vi "EMGain.vi"() -> ()   [LabVIEW 2018]
uses:
  D:/SVN/PM/sdk/AppSamples/LabVIEWSamples/trunk/Release/2018/Dependencies/PVCamNET.dll
  Dependencies/PVCamNET.dll
panel:
  in  "EM Gain Scrollbar":i32(c297)
  in  "Exposure":u32
  in  "?":bool
  out "EM Gain":dbl
  in  "Port":string(combo)
  in  "?":bool
  in  "Gain":string(combo)
  in  "?":bool
  in  "?":bool
  # "EMGain.vi\n\nDescription:\nThis sample code lets the user control the EM Gain.\n\nSteps to run:\n1. Click \"Run\"\n2. Click \"START\"\n3. Update exposure.\n4. Select Port with EM gain enabled\n5. Increase EM Gain\n6. Click \"Start Live\"\n7. Click \"Stop Live\"\n8. Click \"STOP\"\n\nNote: For cameras don't support EM gain this VI shouldn't be run.\nAlso the focus of this VI is to use EM Gain, not Gain and thus Gain is disabled with this VI."
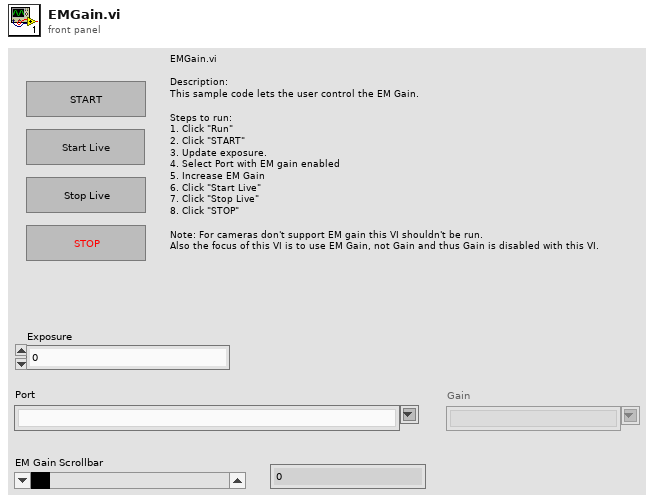
[diagram p1: front panel]
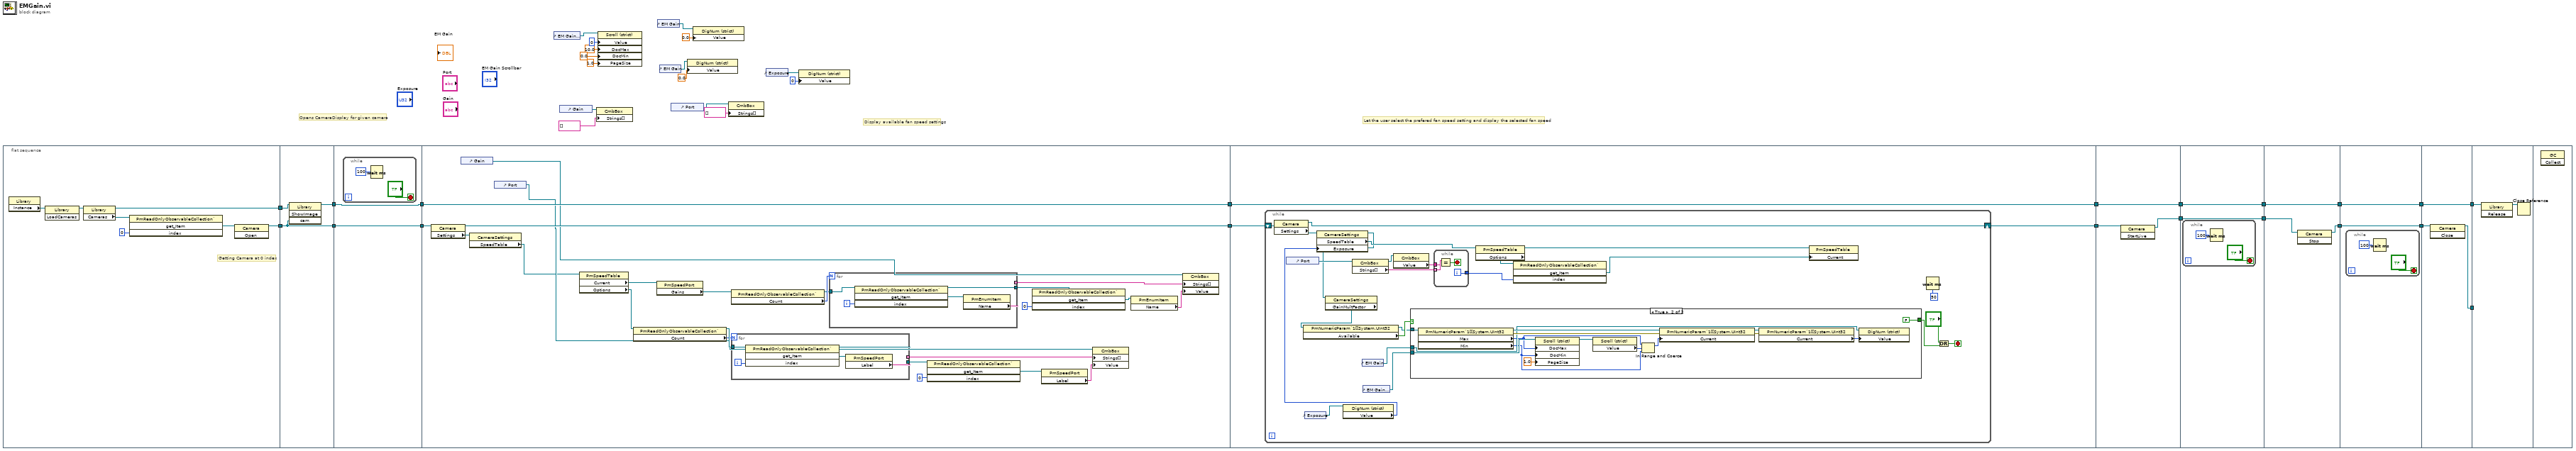
[diagram p0: block diagram]
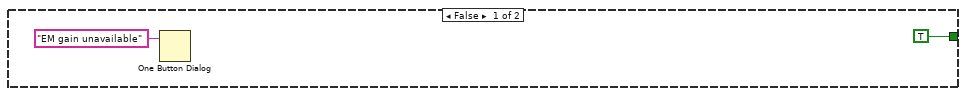
[diagram p2: hidden frame]
diagram:
  # "Let the user select the prefered fan speed setting and display the selected fan speed"
  # "Display available fan speed settings"
  # "Opens CameraDisplay for given camera"
  n1 = flat-sequence {
    tunnel: [w38] -> w35
    tunnel: [w39] -> w34
    tunnel: w35 -> [w45]
    tunnel: w34 -> [w44]
    tunnel: [w44] -> w33
    tunnel: [w43] -> w32
    tunnel: w33 -> [w47]
    tunnel: [w47] -> w30
    tunnel: w32 -> [w46]
    tunnel: [w46] -> w31
    tunnel: [w73] -> w25
    tunnel: [w72] -> w24
    tunnel: w31 -> [w72]
    tunnel: w30 -> [w71]
    tunnel: w25 -> [w86]
    tunnel: [w84] -> w17
    tunnel: w24 -> [w85]
    tunnel: [w85] -> w16
    tunnel: w17 -> [w133]
    tunnel: w16 -> [w134]
    tunnel: [w134] -> w13
    tunnel: [w132] -> w10
    tunnel: w13 -> [w136]
    tunnel: [w136] -> w12
    tunnel: [w135] -> w11
    tunnel: w10 -> [w135]
    tunnel: [w140] -> w15
    tunnel: w12 -> [w141]
    tunnel: [w141] -> w14
    tunnel: w11 -> [w139]
    tunnel: w15 -> [w143]
    tunnel: [w143] -> w27
    tunnel: [w142] -> w26
    tunnel: w14 -> [w142]
    tunnel: w27 -> [w148]
    tunnel: w26 -> [w146]
    tunnel: [w147] -> w29
    tunnel: [w146] -> w28
    tunnel: w29 -> [_]
    tunnel: w28 -> [w150]
    frame #0 {
      # "Getting Camera at 0 index"
      n2 = property class="Library"() -> ("Instance"=w37:refnum<k24>)  [unwired: 2 in, 2 out]
      n3 = invoke class="Library" method="LoadCameras"(reference=w37) -> (reference out=w36:refnum<k24>)  [unwired: 2 in, 2 out]
      n4 = property class="Library"(reference=w36) -> (reference out=w38:refnum<k24>, "Cameras"=w42:refnum<k24>)  [unwired: 1 in, 1 out]
      n5 = invoke class="PmReadOnlyObservableCollection`" method="get_Item"(reference=w42, "index"=0) -> ("get_Item"=w40:refnum<k24>)  [unwired: 2 in, 3 out]
      n6 = invoke class="Camera" method="Open"(reference=w40) -> (reference out=w39:refnum<k24>)  [unwired: 2 in, 2 out]
    }
    frame #1 {
      n7 = invoke class="Library" method="ShowImage"(reference=w45, "cam"=w44) -> (reference out=w43:refnum<k24>)  [unwired: 2 in, 3 out]
    }
    frame #2 {
      n8 = while {
        stop <- "?" stop-if-true
        n9 = Wait (ms)(milliseconds to wait=u32 100) -> ()  [unwired: 1 out]
      }
    }
    frame #3 {
      n10 = property class="Camera"(reference=w71) -> (reference out=w73:refnum<k24>, "Settings"=w70:refnum<k24>)  [unwired: 1 in, 1 out]
      n11 = control-ref of="Gain"() -> (w52:refnum<vi>)
      n12 = property class="CameraSettings"(reference=w70) -> ("SpeedTable"=w50:refnum<k24>)  [unwired: 1 in, 2 out]
      n13 = control-ref of="Port"() -> (w51:refnum<vi>)
      n14 = property class="PmSpeedTable"(reference=w50) -> ("Current"=w69:refnum<k24>, "Options"=w62:refnum<k24>)  [unwired: 1 in, 2 out]
      n15 = property class="PmReadOnlyObservableCollection`"(reference=w62) -> (reference out=w61:refnum<k24>, "Count"=w60:i32)  [unwired: 1 in, 1 out]
      n16 = property class="PmSpeedPort"(reference=w69) -> ("Gains"=w68:refnum<k24>)  [unwired: 1 in, 2 out]
      n17 = property class="PmReadOnlyObservableCollection`"(reference=w68) -> (reference out=w66:refnum<k24>, "Count"=w67:i32)  [unwired: 1 in, 1 out]
      n18 = for {
        N: w60 -> [_]
        tunnel: w61 -> [w78]
        tunnel: [w76] -> w56
        tunnel: [w74] -> w59 mode=indexing
        i -> [w77]
        n19 = invoke class="PmReadOnlyObservableCollection`" method="get_Item"(reference=w78, "index"=w77) -> (reference out=w76:refnum<k24>, "get_Item"=w75:refnum<k24>)  [unwired: 2 in, 2 out]
        n20 = property class="PmSpeedPort"(reference=w75) -> ("Label"=w74:string)  [unwired: 1 in, 2 out]
      }
      n21 = for {
        N: w67 -> [_]
        tunnel: w66 -> [w83]
        tunnel: [w80] -> w64
        tunnel: [w79] -> w63 mode=indexing
        i -> [w82]
        n22 = invoke class="PmReadOnlyObservableCollection`" method="get_Item"(reference=w83, "index"=w82) -> (reference out=w80:refnum<k24>, "get_Item"=w81:refnum<k24>)  [unwired: 2 in, 2 out]
        n23 = property class="PmEnumItem"(reference=w81) -> ("Name"=w79:string)  [unwired: 1 in, 2 out]
      }
      n24 = invoke class="PmReadOnlyObservableCollection`" method="get_Item"(reference=w56, "index"=0) -> ("get_Item"=w57:refnum<k24>)  [unwired: 2 in, 3 out]
      n25 = invoke class="PmReadOnlyObservableCollection`" method="get_Item"(reference=w64, "index"=0) -> ("get_Item"=w65:refnum<k24>)  [unwired: 2 in, 3 out]
      n26 = property class="PmSpeedPort"(reference=w57) -> ("Label"=w58:string)  [unwired: 1 in, 2 out]
      n27 = property class="CmbBox"(reference=w51, "Strings[]"=w59, "Value"=w58) -> ()  [unwired: 1 in, 2 out]
      n28 = property class="PmEnumItem"(reference=w65) -> ("Name"=w55:string)  [unwired: 1 in, 2 out]
      n29 = property class="CmbBox"(reference=w52, "Strings[]"=w63, "Value"=w55) -> ()  [unwired: 1 in, 2 out]
    }
    frame #4 {
      n30 = while {
        shift-right: [w108] -> w84
        shift-left: w86 -> [w109]
        stop <- w90 stop-if-true
        n31 = property class="Camera"(reference=w109) -> (reference out=w108:refnum<k24>, "Settings"=w110:refnum<k24>)  [unwired: 1 in, 1 out]
        n32 = control-ref of="Port"() -> (w99:refnum<vi>)
        n33 = control-ref of="Exposure"() -> (w89:refnum<vi>)
        n34 = property class="DigNum (strict)"(reference=w89) -> ("Value"=w88:u32)  [unwired: 1 in, 2 out]
        n35 = property class="CameraSettings"(reference=w110, "Exposure"=w88) -> (reference out=w97:refnum<k24>, "SpeedTable"=w100:refnum<k24>)  [unwired: 1 in, 1 out]
        n36 = property class="CameraSettings"(reference=w97) -> ("GainMultFactor"=w96:refnum<k24>)  [unwired: 1 in, 2 out]
        n37 = property class="PmNumericParam`1[[System.UInt32"(reference=w96) -> (reference out=w94:refnum<k24>, "Available"=w95:bool)  [unwired: 1 in, 1 out]
        n38 = property class="CmbBox"(reference=w99) -> (reference out=w102:refnum<vi>, "Strings[]"=w106:string[])  [unwired: 1 in, 1 out]
        n39 = control-ref of="EM Gain"() -> (w93:refnum<vi>)
        n40 = control-ref of="EM Gain Scrollbar"() -> (w87:refnum<vi>)
        n41 = property class="CmbBox"(reference=w102) -> ("Value"=w101:string)  [unwired: 1 in, 2 out]
        n42 = case shown="True" w95 {
          tunnel: w94 -> [_ w127]
          tunnel: w93 -> [_ w119]
          tunnel: [TRUE FALSE] -> w91
          tunnel: w87 -> [_ w118]
          frame False {
            n43 = One Button Dialog(message="EM gain unavailable") -> ()  [unwired: 1 in, 1 out]
          }
          frame True {
            n44 = property class="PmNumericParam`1[[System.UInt32"(reference=w127) -> (reference out=w125:refnum<k24>, error out=w123:errorcluster, "Max"=w117:u32, "Min"=w116:u32)  [unwired: 1 in]
            n45 = property class="Scroll (strict)"(reference=w118, "DocMax"=w117, "DocMin"=w116, "PageSize"=1.0 ("Page Size")) -> (reference out=w114:refnum<vi>)  [unwired: 1 in, 1 out]
            n46 = property class="Scroll (strict)"(reference=w114) -> ("Value"=w113:i32)  [unwired: 1 in, 2 out]
            n47 = In Range and Coerce(upper limit=w117, x=w113, lower limit=w116) -> (coerced(x)=w126:u32)  [unwired: 1 out]
            n48 = property class="PmNumericParam`1[[System.UInt32"(reference=w125, error in=w123, "Current"=w126) -> (reference out=w124:refnum<k24>, error out=w122:errorcluster)
            n49 = property class="PmNumericParam`1[[System.UInt32"(reference=w124, error in=w122) -> ("Current"=w121:u32)  [unwired: 2 out]
            n50 = property class="DigNum (strict)"(reference=w119, "Value"=w121) -> ()  [unwired: 1 in, 2 out]
          }
        }
        n51 = while {
          tunnel: w106 -> [w131] mode=indexing
          tunnel: [w129] -> w104
          tunnel: w101 -> [w128]
          i -> [w129]
          stop <- w130 stop-if-true
          n52 = Equal?(x=w131, y=w128) -> (x = y?=w130:bool)
        }
        n53 = property class="PmSpeedTable"(reference=w100) -> (reference out=w103:refnum<k24>, "Options"=w105:refnum<k24>)  [unwired: 1 in, 1 out]
        n54 = invoke class="PmReadOnlyObservableCollection`" method="get_Item"(reference=w105, "index"=w104) -> ("get_Item"=w98:refnum<k24>)  [unwired: 2 in, 3 out]
        n55 = property class="PmSpeedTable"(reference=w103, "Current"=w98) -> ()  [unwired: 1 in, 2 out]
        n56 = Wait (ms)(milliseconds to wait=u32 50) -> ()  [unwired: 1 out]
        n57 = Or(x="?", y=w91) -> (x .or. y?=w90:bool)
      }
    }
    frame #5 {
      n58 = invoke class="Camera" method="StartLive"(reference=w133) -> (reference out=w132:refnum<k24>)  [unwired: 2 in, 2 out]
    }
    frame #6 {
      n59 = while {
        stop <- "?" stop-if-true
        n60 = Wait (ms)(milliseconds to wait=u32 100) -> ()  [unwired: 1 out]
      }
    }
    frame #7 {
      n61 = invoke class="Camera" method="Stop"(reference=w139) -> (reference out=w140:refnum<k24>)  [unwired: 2 in, 2 out]
    }
    frame #8 {
      n62 = while {
        stop <- "?" stop-if-true
        n63 = Wait (ms)(milliseconds to wait=u32 100) -> ()  [unwired: 1 out]
      }
    }
    frame #9 {
      n64 = invoke class="Camera" method="Close"(reference=w148) -> (reference out=w147:refnum<k24>)  [unwired: 2 in, 2 out]
    }
    frame #10 {
      n65 = invoke class="Library" method="Release"(reference=w150) -> (reference out=w149:refnum<k24>)  [unwired: 2 in, 2 out]
      n66 = Close Reference(reference=w149) -> ()  [unwired: 1 in, 1 out]
    }
    frame #11 {
      n67 = invoke class="GC" method="Collect"() -> ()  [unwired: 3 in, 3 out]
    }
  }
  n68 = control-ref of="EM Gain Scrollbar"() -> (w7:refnum<vi>)
  n69 = control-ref of="Gain"() -> (w23:refnum<vi>)
  n70 = property class="CmbBox"(reference=w23, "Strings[]"=string[] [] ("Strings []")) -> ()  [unwired: 1 in, 2 out]
  n71 = property class="Scroll (strict)"(reference=w7, "Value"=0, "DocMax"=10.0 ("Doc Max"), "DocMin"=0.0 ("Doc Min"), "PageSize"=1.0 ("Page Size")) -> ()  [unwired: 1 in, 2 out]
  n72 = control-ref of="EM Gain"() -> (w2:refnum<vi>)
  n73 = control-ref of="EM Gain"() -> (w19:refnum<vi>)
  n74 = control-ref of="Port"() -> (w21:refnum<vi>)
  n75 = property class="DigNum (strict)"(reference=w19, "Value"=0.0) -> ()  [unwired: 1 in, 2 out]
  n76 = property class="DigNum (strict)"(reference=w2, "Value"=0.0) -> ()  [unwired: 1 in, 2 out]
  n77 = property class="CmbBox"(reference=w21, "Strings[]"=string[] [] ("Strings []")) -> ()  [unwired: 1 in, 2 out]
  n78 = control-ref of="Exposure"() -> (w9:refnum<vi>)
  n79 = property class="DigNum (strict)"(reference=w9, "Value"=u32 0) -> ()  [unwired: 1 in, 2 out]
